vi "chunkify.vi"(11 "String":string="Late in the nineteenth century Sweden was a quite underdeveloped and poor country. One thing that the Swedes did have though, was raw materials. And one of the most prosperous industries in late 1870:ies was something that became, and still is, very important to IKEA; The wood industry. \nHowever, in 1879 there was a recession and the sawmill owners in Sundsvall in northern Sweden could not sell their sawed timber. So, they cut the wages of the saw mill workers. The workers protested and decided to not go to the mills. But the military was called in to force them back to work. This quite dramatic event, the Sundsvall strike, marked the start of the developing of unions in Sweden.\nUnions were developed to protect the rights of workers, but it was a bumpy road. Even some fifty years later, Sweden had the highest number of labour market conflict days among the countries in Europe. At that point, Sweden was at a crossroads. Some system needed to be put in place to negotiate between the interests of the employers and employees, without strikes and lockouts.\nOne way to go, perhaps the most common today, would be to put more labour market legislation in place. Write more laws. For instance laws dictating in what situations a strike is legitimate. Parliament would be a kind of go-between employers and employees and try to find a middle ground. That would also mean that changes in the political landscape could impact the labour laws.\nThe other way, would be for organisations representing employers and employees to take it upon themselves to create binding agreements on the most important issues in their interests. That means a joint responsibility for developing regulations of the labour market. \nA decision to take the second option was made in the agreement signed in 1938 by the Swedish trade union Confederation and the Federation of Swedish Industry in Saltsjöbaden outside Stockholm, marking the birth of the Swedish model.\nThis concept of letting the unions and employer organisations determine the terms and conditions for employment in Sweden, without interference from the government is a key concept in Swedish labour law. So we will look at that in detail soon.\nBut first let's have a quick look at how things work in many other places, And what it looked like in Sweden before the Saltjöbaden Agreement.\n") -> (3 "Chunks":string[](array[string]))   [LabVIEW 2018]
uses:
  <vilib>/regexp/Match Regular Expression.xnode
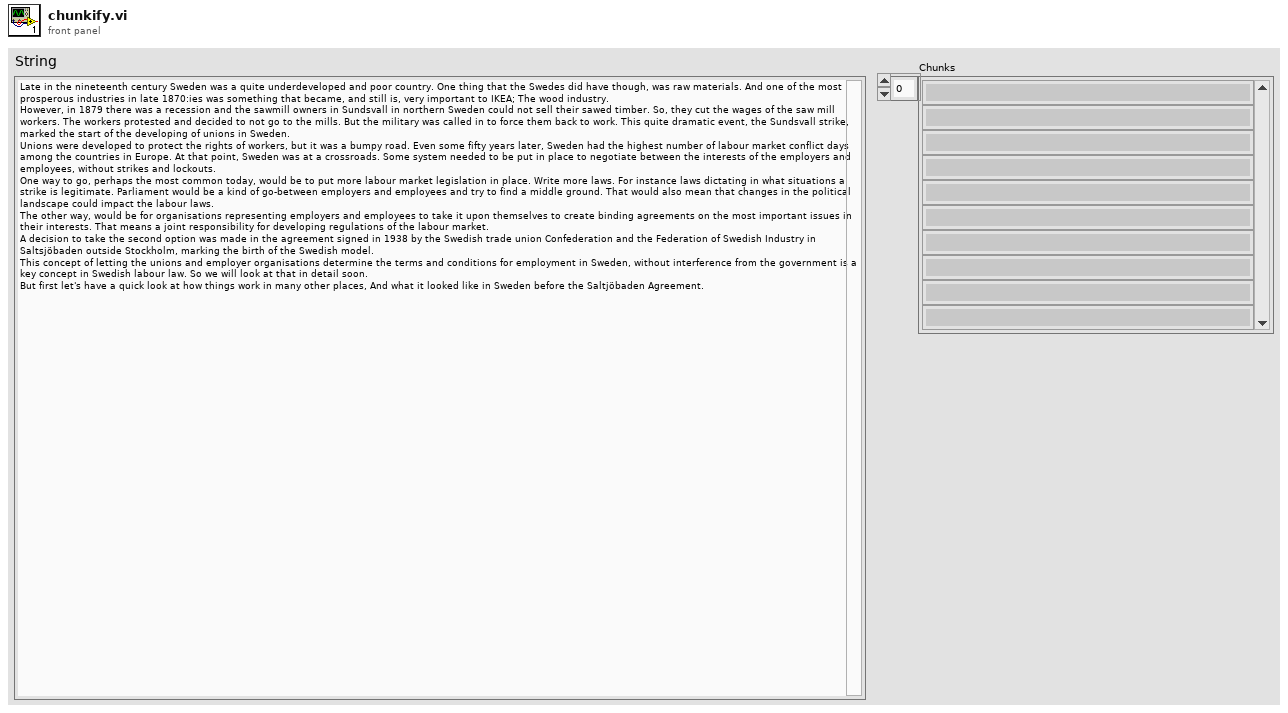
[diagram p1: front panel]
types:
  T1 = cluster{"Font Name:":string, "Size":i16, "Strikeout?":bool, "Italic?":bool, "Underline?":bool, "Outline?":bool, "Shadow?":bool, "Bold?":bool}
  T2 = cluster{"left":i16, "top":i16, "right":i16, "bottom":i16}
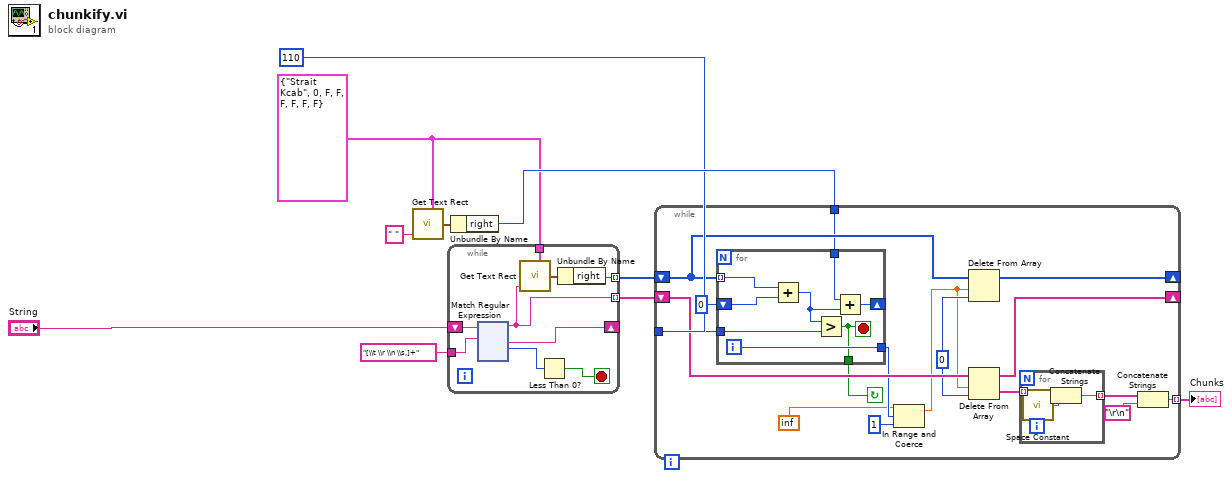
[diagram p0: block diagram]
diagram:
  w3 = T1 {"Font Name:"="Strait Kcab", "Size"=0, "Strikeout?"=FALSE, "Italic?"=FALSE, "Underline?"=FALSE, "Outline?"=FALSE, "Shadow?"=FALSE, "Bold?"=FALSE} ("[user-specified font]")
  n1 = call <vilib>:"Get Text Rect.vi"("text"=" ", "[user-specified font]"=w3) -> ("rect"=w9:T2)  [unwired: 7 in]
  n2 = while {
    shift-right: [w18] -> _
    shift-left: "String" -> [w19]
    tunnel: [w14] -> w6 mode=indexing
    tunnel: [w13] -> w7 mode=indexing
    tunnel: w3 -> [w12]
    tunnel: "[\\t \\r \\n \\s,]+" ("regular expression") -> [w11]
    stop <- w15 stop-if-true
    n3 = xnode "Match Regular Expression"("input string"=w19, "regular expression"=w11) -> ("before match"=w13:string, "after match"=w18:string, "offset past match"=w16:i32)  [unwired: 4 in, 2 out]
    n4 = call <vilib>:"Get Text Rect.vi"("text"=w13, "[user-specified font]"=w12) -> ("rect"=w17:T2)  [unwired: 7 in]
    n5 = Less Than 0?(x=w16) -> (x < 0?=w15:bool)
    n6 = Unbundle By Name(w17) -> ("right"=w14:i16)
  }
  n7 = Unbundle By Name(w9) -> ("right"=w4:i16)
  n8 = while {
    shift-right: [w148] -> _
    shift-left: w6 -> [w149]
    shift-right: [w146] -> _
    shift-left: w7 -> [w147]
    tunnel: [w141] -> w5 mode=indexing
    tunnel: w4 -> [w139]
    tunnel: i16 110 ("y") -> [w138]
    stop <- w140 continue-if-true
    w145 = 0 ("index")
    n9 = for {
      tunnel: w149 -> [w158] mode=indexing
      shift-right: [w153] -> _
      shift-left: i16 0 -> [w157]
      tunnel: [w155] -> w136
      tunnel: [w154] -> w140
      tunnel: w139 -> [w152]
      tunnel: w138 -> [w151]
      i -> [w155]
      stop <- w154 stop-if-true
      n10 = Add(x=w158, y=w157) -> (x+y=w156:i16)
      n11 = Greater?(x=w156, y=w151) -> (0:w154:bool)
      n12 = Add(x=w152, y=w156) -> (x+y=w153:i16)
    }
    n13 = In Range and Coerce(upper limit=inf, x=w136, lower limit=1) -> (coerced(x)=w135:dbl)  [unwired: 1 out]
    n14 = Delete From Array(array=w149, length=w135, index=w145) -> (array with subset deleted=w148:i16[])  [unwired: 1 out]
    n15 = Delete From Array(array=w147, length=w135, index=w145) -> (deleted portion=w144:string[], array with subset deleted=w146:string[])
    n16 = for {
      tunnel: w144 -> [w161] mode=indexing
      tunnel: [w160] -> w143 mode=indexing
      n17 = call <vilib>:"Space Constant.vi"() -> ("String"=w159:string)
      n18 = Concatenate Strings(w161, w159) -> (w160:string)
    }
    n19 = Concatenate Strings(w143, "\r\n") -> (w141:string)
  }
  "Chunks" <- w5
